vi "CSGaussmeter.remove services.vi"(0 "i ref in":refnum<vi>, 7 "ms timeout (10000)":i32=10000, 11 "error in (no error)":errorcluster) -> (4 "i ref out":refnum<vi>, 8 "timed out":bool, 15 "error out":errorcluster)   [LabVIEW 2014, in "CSGaussmeter.lvlib"]
uses:
  CSGaussmeter.lvlib
  CSlibraries-extern/DimLVEvent/LVDimInterface/LVDimInterface.lvlib
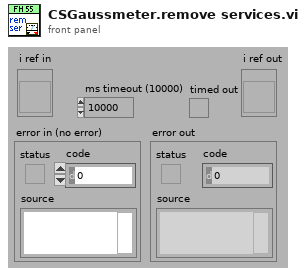
[diagram p1: front panel]
types:
  T1 = typedef "CSGaussmeter.lvlib/CSGaussmeter.i attribute.ctl" = cluster{"Name":string, "VISA Resource Name":refnum<visa-resource-name>, "actValues":cluster{" Limit":bool, "Unit ":T2, "Temp_Unit":T3, "Max":T4, " Filter":bool, " Peak":bool, " Auto_Range":bool, "Range":T5, " Rel":bool, " CTemp":bool, " CField":bool, "AC_DC ":bool, "Set_lower":cluster{"Numeric":dbl, "Cancel Button":bool, "Unit":T6}, "Set_upper":cluster{"Numeric":dbl, "Cancel Button":bool, "Unit":T6}, "Set_Rel":cluster{"Numeric":dbl, "Cancel Button":bool, "Unit":T6}, "Zero":bool, " Local":bool, "Reset":bool, " Init":bool}, "FH 55 Gauss-/Teslameter":T7, "MAX_Value":T8, "MIN_Value":T8, "Rel_Value":T8, "Array ":string[], "LIMU":dbl, " LIML":dbl, "Messwerte 2":string, "Messwerte ":cluster{"Numeric":i32, "OK Button":bool}, "serviceID":cluster{"Current ID":i32, "Unit ID":i32, "Temp ID":i32, "Name ID \n":i32, "Visa ID ":i32}, "setValues ":cluster{" Limit":bool, "Unit ":T2, "Temp_Unit":T3, "Max":T4, " Filter":bool, " Peak":bool, " Auto_Range":bool, "Range":T5, " Rel":bool, " CTemp":bool, " CField":bool, "AC_DC ":bool, "Set_lower":cluster{"Numeric":dbl, "Cancel Button":bool, "Unit":T6}, "Set_upper":cluster{"Numeric":dbl, "Cancel Button":bool, "Unit":T6}, "Set_Rel":cluster{"Numeric":dbl, "Cancel Button":bool, "Unit":T6}, "Zero":bool, " Local":bool, "Reset":bool, " Init":bool}}
  T2 = typedef "FH 55.lvlib/Unit.ctl" = enum16{"T", "G", "A/m"}
  T3 = typedef "FH 55.lvlib/Temp_Unit.ctl" = enum16{"Temp off", "Celsius", "Fahrenheit"}
  T4 = typedef "FH 55.lvlib/Max.ctl" = enum16{"MAX off", "Show MAX", "MAX/MIN"}
  T5 = typedef "FH 55.lvlib/Range.ctl" = enum16{"1", "2", "3", "4", "5", "6", "7"}
  T6 = typedef "FH 55.lvlib/Unit2.ctl" = enum16{"mT", "G", "kA/m"}
  T7 = typedef "FH 55.lvlib/Display.ctl" = cluster{"current value":string, "Limit":string, "Remote":string, "function ":string, "Cluster":cluster{"AC/DC":string, "Auto":string, "Filter":string, "Range":string, "Rel":string, "Peak":string}}
  T8 = typedef "FH 55.lvlib/Value_String.ctl" = cluster{"Numeric":dbl, "String":string}
  T9 = cluster{"Current ID":i32, "Unit ID":i32, "Temp ID":i32, "Name ID":i32, "Visa ID":i32}
  T10 = cluster{"Current ID":i32, "Unit ID":i32, "Temp ID":i32, "Name ID \n":i32, "Visa ID ":i32}
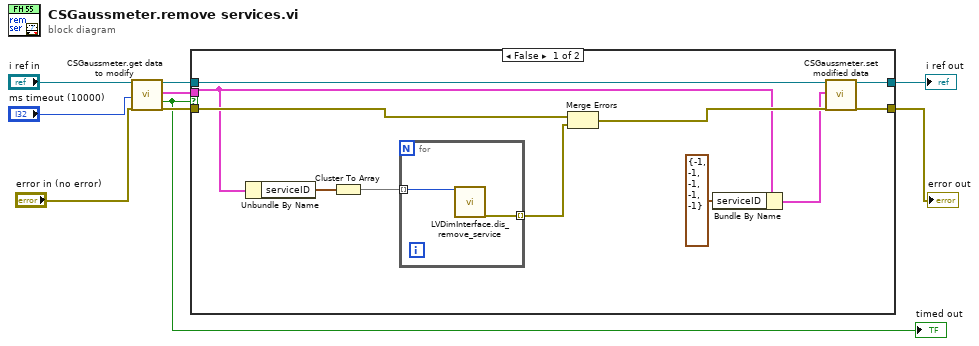
[diagram p0: block diagram]
diagram:
  n1 = call "CSGaussmeter.get data to modify.vi"("i ref in"="i ref in", "ms timeout (10000)"="ms timeout (10000)", "error in (no error)"="error in (no error)") -> ("i ref out"=w6:refnum<vi>, "i attribute"=w5:T1, "timed out"=w1:bool, "error out"=w4:errorcluster)  [unwired: 13 in]
  "timed out" <- w1
  n2 = case shown="False" w1 {
    tunnel: w6 -> [w16 w23]
    tunnel: w5 -> [w10 _]
    tunnel: w4 -> [w18 w24]
    tunnel: [w14 w23] -> w3
    tunnel: [w13 w24] -> w2
    frame False {
      n3 = Unbundle By Name(w10) -> ("serviceID"=w20:T10)
      n4 = Cluster To Array(cluster=w20) -> (array=w19:i32[])
      n5 = for {
        tunnel: w19 -> [w22] mode=indexing
        tunnel: [w21] -> w17 mode=indexing
        n6 = call "LVDimInterface.dis_remove_service.vi"("my_serviceID"=w22) -> ("error out"=w21:errorcluster)  [unwired: 18 in]
      }
      n7 = Merge Errors(w18, w17) -> (w15:errorcluster)
      n8 = Bundle By Name(cluster=w10, "serviceID"=T9 {"Current ID"=-1, "Unit ID"=-1, "Temp ID"=-1, "Name ID"=-1, "Visa ID"=-1}) -> (w12:T1)
      n9 = call "CSGaussmeter.set modified data.vi"("i ref in"=w16, "i attribute"=w12, "error in (no error)"=w15) -> ("i ref out"=w14:refnum<vi>, "error out"=w13:errorcluster)  [unwired: 15 in]
    }
    frame True {
    }
  }
  "error out" <- w2
  "i ref out" <- w3
